vi "PID-position control.vi"() -> ()   [LabVIEW 2018]
uses:
  <vilib>/Platform/TimedLoop/XDataNode/timing_clust.ctl
  <vilib>/Platform/TimedLoop/XDataNode/nitl_modes.ctl
  <vilib>/Platform/TimedLoop/XDataNode/wakeup.ctl
  <vilib>/FPGAPlugInAG/myRIO-1900/niLvFpga_Open_myRIO-1900.vi
  <vilib>/rvi/interface/common/dynamic/niFpgaDynamicAddResources.vi
  <vilib>/Utility/error.llb/Error Cluster From Error Code.vi
  <vilib>/rvi/errors/niLvFpgaAdjustHostInterfaceError.vi
  <vilib>/rvi/interface/nirviOpenFPGA/nirviOpenFPGA.xnode
  FPGA Bitfiles/Dentalrobot_FPGATarget_FPGADentalroboto_PTkoih3chUc.lvbitx
  FPGA/FPGA_myRIO.vi
  <vilib>/rvi/interface/nirviReadWriteControl/nirviReadWriteControl.xnode
  <vilib>/Platform/TimedLoop/XDataNode/XDataNode.xnode
  <vilib>/Platform/TimedLoop/XDataNode/XDNodeRunTimeDep.lvlib
  <vilib>/rvi/interface/Simulation/niFpgaSimulationCallBeginRW.vi
  NiFpgaLv.dll
panel:
  out "Duty Cycle (Abs)":dbl
  in  "Desired position":i32 step=10000
  in  "PID Gains":cluster{"Kp":dbl, "Kd":dbl, "Ki":dbl}={"Kp"=0.002, "Kd"=0.007, "Ki"=9e-05} {"Kp" step=0.001 format="%#_8f"; "Kd" step=0.01; "Ki" format="%#_6f"}
  out "error out":errorcluster
  out "JumpBy2Error 4":i16
  out "Waveform Chart":i32(graph)
  in  "stop":bool
  out "Position4":i32
  in  "Reset 4":bool
  in  "DIR4":bool
  in  "ENA4":bool
  out "finished late":dbl
  # "275:1   140800\n67:1      34304"
  # "rpm"
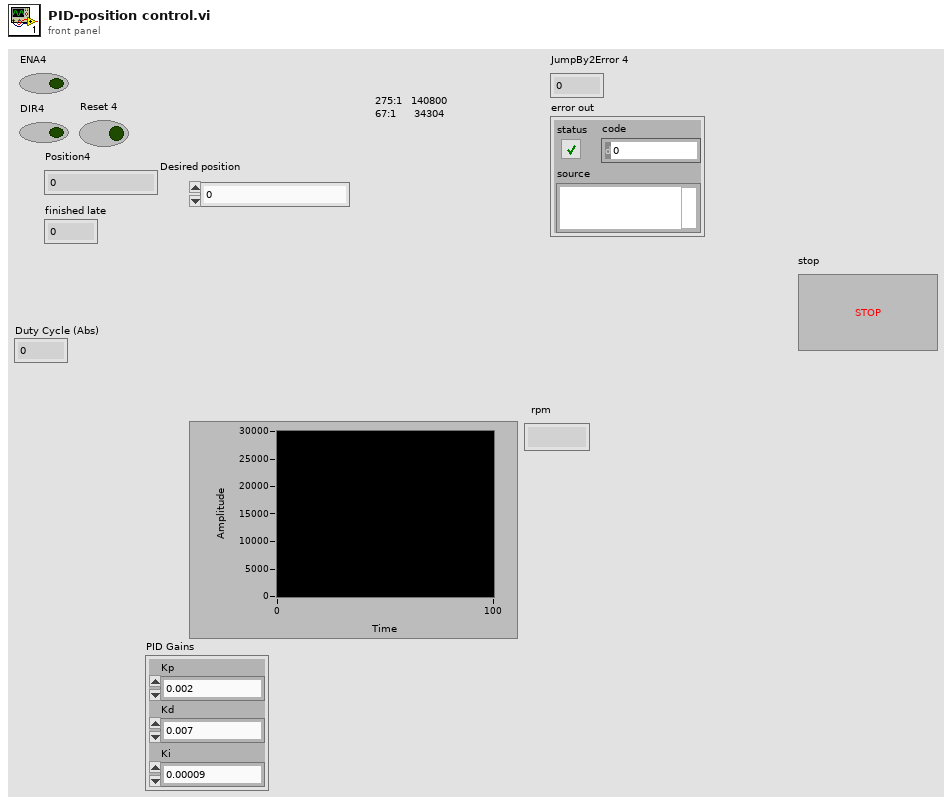
[diagram p1: front panel]
types:
  T1 = typedef "XDNodeRunTimeDep.lvlib/timing_clust.ctl" = cluster{"Expected End [f-1]":u64, "Actual End [f-1]":u64, "Finished Late? [f-1]":bool, "Expected End [i-1]":u64, "Actual End [i-1]":u64, "Finished Late? [i-1]":bool, "Expected Start [i]":u64, "Actual Start [i]":u64, "Expected Start [f]":u64, "Actual Start [f]":u64, "Source Name":string, "Structure Name":string, "Period":i64, "Deadline":i64, "Offset":i64, "Start":i64, "Priority":i32, "Timeout":i32, "Mode":T2, "Wakeup Reason":T3, "Error":errorcluster, "Source Type":string, "Secondary Source Type":string, "Global End Time":u64, "Global Start Time":u64, "Frame Duration":u64, "Iteration Duration":u64, "Assigned CPU":i32, "I/O Scan Engine Mode":u32}
  T2 = typedef "XDNodeRunTimeDep.lvlib/nitl_modes.ctl" = enum32{"No Change", "Process missed periods, maintain original phase", "Discard missed periods, maintain original phase", "Process missed periods, ignore original phase", "Discard missed periods, ignore original phase"}
  T3 = typedef "XDNodeRunTimeDep.lvlib/wakeup.ctl" = enum32{"Normal", "Aborted", "Asynchronous wakeup", "Timing source error", "Timed loop error", "Timeout"}
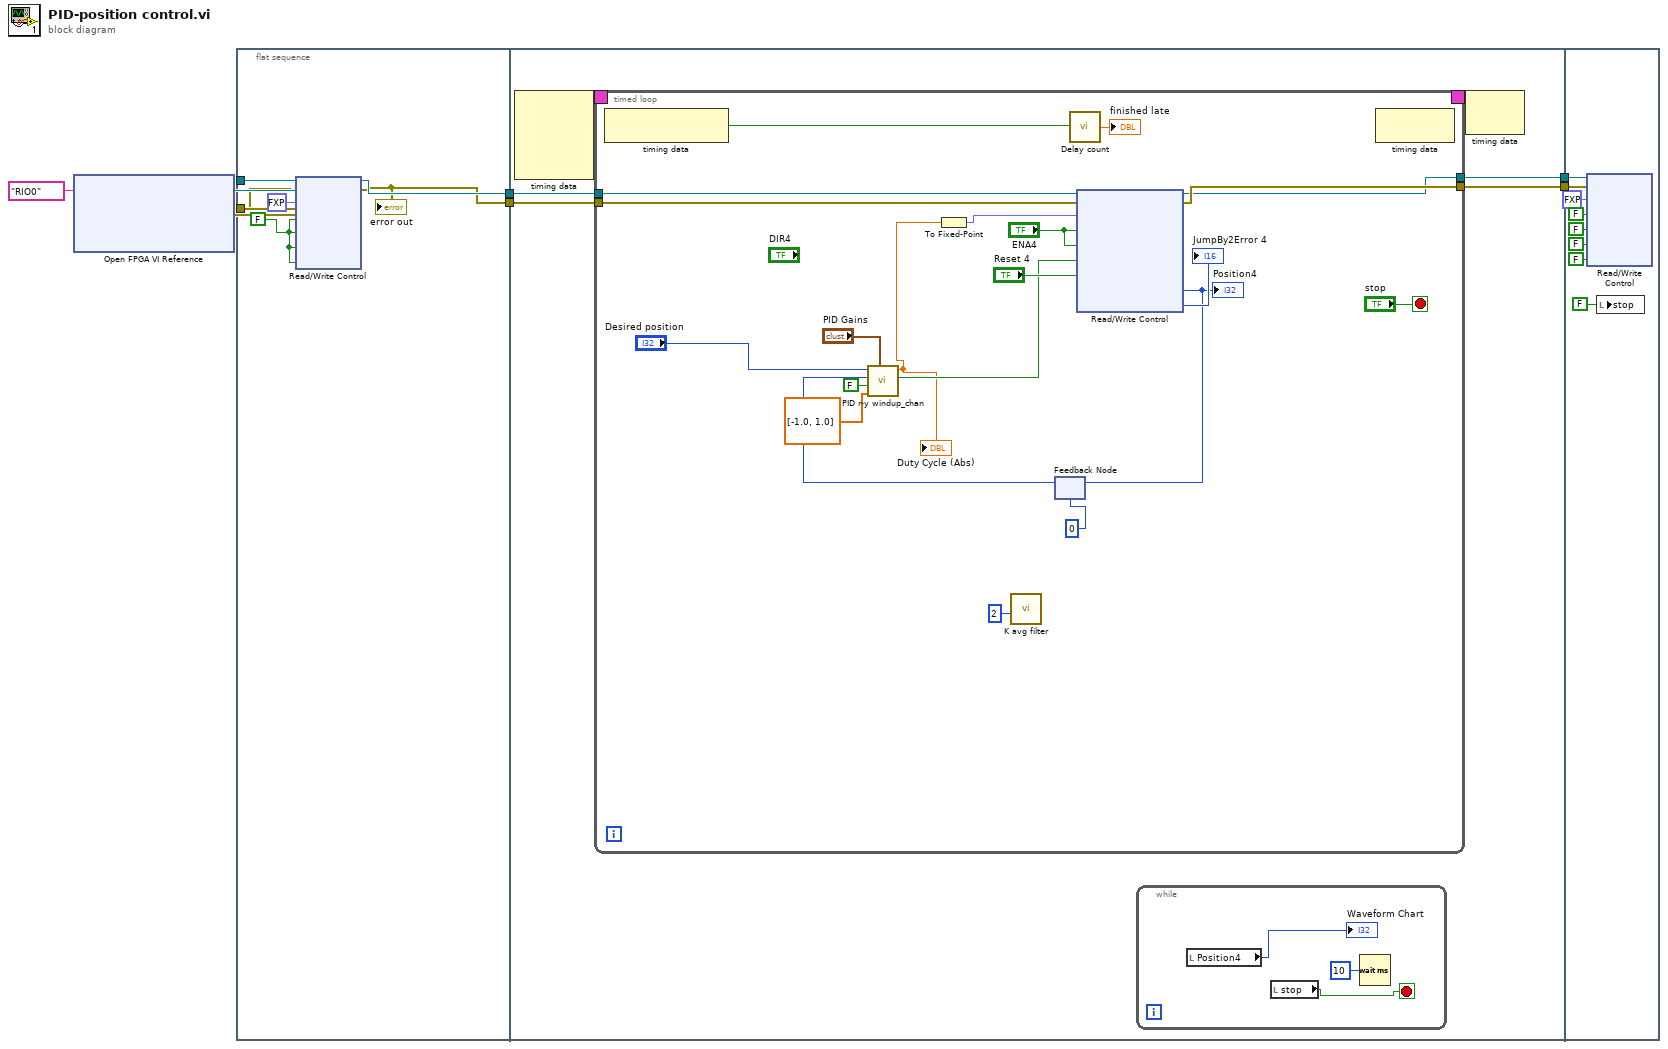
[diagram p0: block diagram]
diagram:
  n1 = xnode "Open FPGA VI Reference"("resource name"=tag "RIO0") -> ("FPGA VI Reference Out"=w3:refnum<k20>, "error out"=w2:errorcluster)  [unwired: 1 in]
  n2 = flat-sequence {
    tunnel: [w11] -> w7
    tunnel: [w10] -> w6
    tunnel: w3 -> [w9]
    tunnel: w2 -> [w8]
    tunnel: w7 -> [w14]
    tunnel: w6 -> [w15]
    tunnel: [w17] -> w5
    tunnel: [w16] -> w4
    tunnel: w5 -> [w56]
    tunnel: w4 -> [w55]
    frame #0 {
      w13 = FALSE
      n3 = xnode "Read/Write Control"("FPGA VI Reference In"=w9, "error in"=w8, "CH4 DC"=fxp<+,32,0> 0.0, "ENA4"=w13, "STBY4"=w13, "DIR4"=w13, "Reset 4"=w13) -> ("FPGA VI Reference Out"=w11:refnum<k20>, "error out"=w10:errorcluster)
      "error out" <- w10
    }
    frame #1 {
      n4 = node-c288() -> (w19:T1)  [unwired: 4 in]
      n5 = timed-loop {
        timing: w19 -> [_]
        timing-out: [_] -> w18
        tunnel: w14 -> [w43]
        tunnel: w15 -> [w42]
        tunnel: [w34] -> w17
        tunnel: [w35] -> w16
        stop <- "stop" stop-if-true
        n6 = node-c288() -> (w41:bool)  [unwired: 1 in]
        n7 = call "K avg filter.vi"("num avg"=2) -> ()  [unwired: 10 in, 1 out]
        n8 = feedback #1(0) -> (w26:i32)
        n9 = call "PID r-y windup_chan.vi"("PID Gains"="PID Gains", "Saturation"=dbl[] [-1.0, 1.0], "Reverse Motor?"=FALSE, "Encoder position"=w26, "Reference"="Desired position") -> ("DIR"=w25:bool, "Duty Cycle (Abs)"=w23:dbl)  [unwired: 3 in, 2 out]
        "Duty Cycle (Abs)" <- w23
        n10 = To Fixed-Point(number=w23) -> (fixed-point=w32:fxp<+/-,32,16>)  [unwired: 1 in]
        n11 = call "Delay count.vi"("Finished Late? [i-1]"=w41) -> ("Count"=→"finished late":dbl)
        n12 = xnode "Read/Write Control"("FPGA VI Reference In"=w43, "error in"=w42, "CH4 DC"=w32, "ENA4"="ENA4", "STBY4"="ENA4", "DIR4"=w25, "Reset 4"="Reset 4") -> ("FPGA VI Reference Out"=w34:refnum<k20>, "error out"=w35:errorcluster, "Position4"=w27:i32, "JumpBy2Error 4"=→"JumpBy2Error 4":i16)
        "Position4" <- w27
        n13 = feedback-in #1(w27) -> ()
        n14 = node-c288() -> ()  [unwired: 1 in, 1 out]
      }
      n15 = while {
        stop <- w21 stop-if-true
        n16 = local read "Position4"() -> (→"Waveform Chart":i32)
        n17 = local read "stop"() -> (w21:bool)
        n18 = Wait (ms)(milliseconds to wait=u32 10) -> ()  [unwired: 1 out]
      }
      n19 = node-c288(w18) -> ()  [unwired: 1 out]
    }
    frame #2 {
      n20 = xnode "Read/Write Control"("FPGA VI Reference In"=w56, "error in"=w55, "CH4 DC"=fxp<+,32,0> 0.0, "ENA4"=FALSE, "STBY4"=FALSE, "DIR4"=FALSE, "Reset 4"=FALSE) -> ()  [unwired: 2 out]
      n21 = local write "stop"(FALSE ("stop")) -> ()
    }
  }
